vi "PH_Cam_BaseClass.set modified data.vi"(0 "i ref in":refnum<vi>, 2 "i attribute":T1={"Gui Refs"={"Frame Rate"=refnum, "Get Frame Rate"=refnum, "Show Image"=refnum, "Get Histogram"=refnum, "Mapping"=refnum, "Histogram"=refnum, "Center Cross"=refnum, "Center of Gravity"=refnum, "Scale Factor [%]"=refnum, "Save Image"=refnum, "Palette"=refnum, "Subtract Background"=refnum, "Cam Error"=refnum, "On"=refnum, "Cam List"=refnum}, "Cam"={"Source Notifier"=refnum, "Error"={"status"=FALSE, "code"=0, "source"=""}, "Camera ID"="N/A"}, "Images"={"Cam"=refnum, "Operation"=refnum, "PSDB"=refnum}, "Window Image"={"Indicate Image"=FALSE, "Window No."=0, "Scale Facor"=0.5, "Center Cross"=FALSE, "Subtract Backgr"=FALSE, "CoG"=FALSE, "Color Palette"=[], "Image On"=FALSE}, "Default Prdc Int"=50, "Performance"={"on"=FALSE, "Timestamp Last Frame"=0}, "Histogram"={"on"=FALSE, "Mapping"=FALSE}, "Save Image"={"Save"=FALSE, "File refnum"=refnum}, "Setting Service ID"=0, "Screen"={"x-resolution"=0, "y-resolution"=0}, "On"=FALSE, "Constructor finished"=FALSE, "configured"=FALSE} {"Cam"."Error"."code" format="%.0x"}, 5 "error in (no error)":errorcluster) -> (14 "i ref out":refnum<vi>, 19 "error out":errorcluster)   [LabVIEW 2014, in "PH_Cam_BaseClass.lvlib"]
doc: "Writes the data into the attribute of an object. Then, the attribute dara are unlocked using the \"release\" method. Prior to calling THIS method, the attribute data must have been locked using the methods \"lock\" or \"get data to modify\".\n\n\nLicense Agreement for this software:\n\nCopyright (C)\nGesellschaft für Schwerionenforschung, GSI\nPlanckstr. 1\n64291 Darmstadt\nGermany\n\nContact: D.Beck@gsi.de \n\nThis program is free software; you can redistribute it and/or modify it under the terms of the GNU General Public License as published by the Free Software Foundation; either version 2 of the license, or (at your option) any later version.\n\nThis program is distributed in the hope that it will be useful, but WITHOUT ANY WARRANTY; without even the implied warranty of MERCHANTABILITY or FITNESS FOR A PARTICULAR PURPOSE. See the GNU General License for more details (http://www.gnu.org).\n\nGesellschaft für Schwerionenforschung, GSI\nPlanckstr. 1, 64291 Darmstadt, Germany\nFor all questions and ideas contact: M.Richter@gsi.de, H.Brand@gsi.de or D.Beck@gsi.de.\nLast update: 17-JUN-2004"
uses:
  PH_Cam_BaseClass.lvlib
  PH_Cam_BaseClass.i attribute.ctl
  PH_Cam_BaseClass.GUI Refs.ctl
  <vilib>/vision/Image Controls.llb/IMAQ Image.ctl
  CSCore/CSObj/CSObj.lvlib
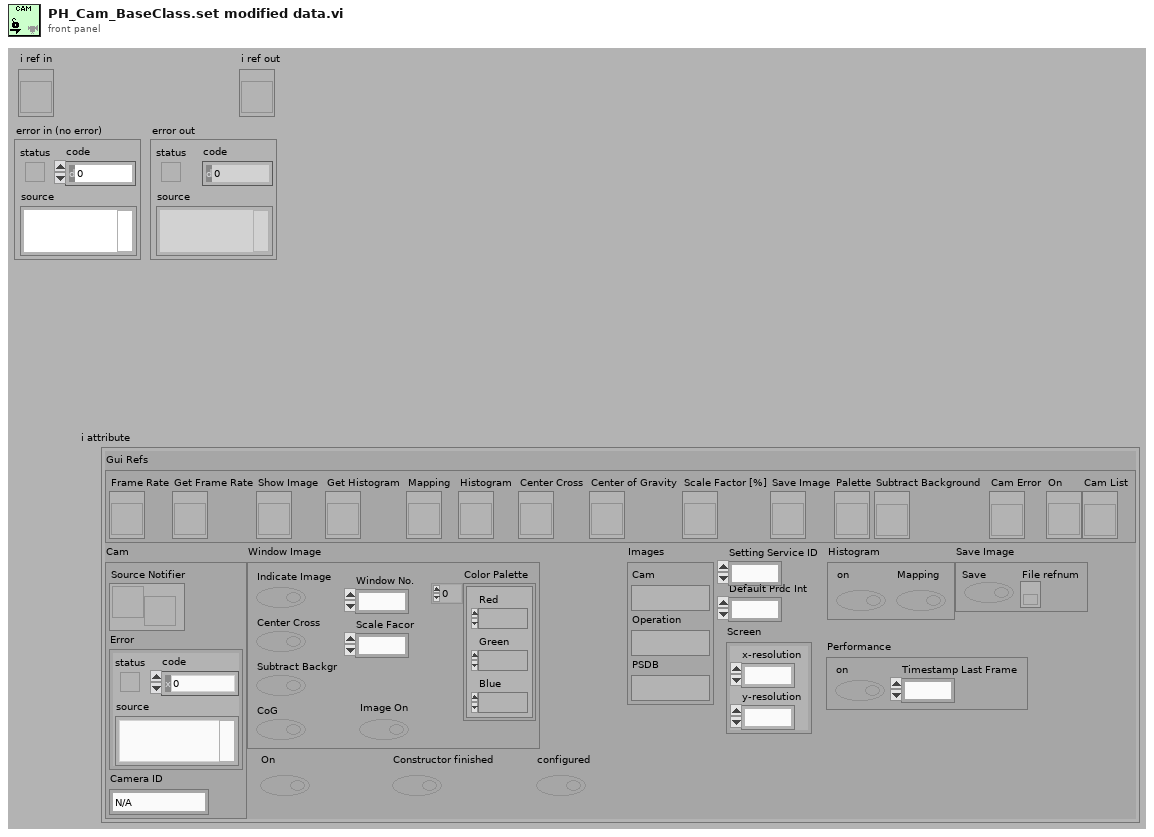
[diagram p1: front panel]
types:
  T1 = typedef "PH_Cam_BaseClass.lvlib/PH_Cam_BaseClass.i attribute.ctl" = cluster{"Gui Refs":T2, "Cam":cluster{"Source Notifier":refnum<notifier>, "Error":errorcluster, "Camera ID":string}, "Images":cluster{"Cam":T3, "Operation":T3, "PSDB":T3}, "Window Image":cluster{"Indicate Image":bool, "Window No.":i32, "Scale Facor":dbl, "Center Cross":bool, "Subtract Backgr":bool, "CoG":bool, "Color Palette":cluster{"Red":u8, "Green":u8, "Blue":u8}[], "Image On":bool}, "Default Prdc Int":i32, "Performance":cluster{"on":bool, "Timestamp Last Frame":i32}, "Histogram":cluster{"on":bool, "Mapping":bool}, "Save Image":cluster{"Save":bool, "File refnum":refnum<file>}, "Setting Service ID":i32, "Screen":cluster{"x-resolution":i16, "y-resolution":i16}, "On":bool, "Constructor finished":bool, "configured":bool}
  T2 = typedef "PH_Cam_BaseClass.lvlib/PH_Cam_BaseClass.GUI Refs.ctl" = cluster{"Frame Rate":refnum<vi>, "Get Frame Rate":refnum<vi>, "Show Image":refnum<vi>, "Get Histogram":refnum<vi>, "Mapping":refnum<vi>, "Histogram":refnum<vi>, "Center Cross":refnum<vi>, "Center of Gravity":refnum<vi>, "Scale Factor [%]":refnum<vi>, "Save Image":refnum<vi>, "Palette":refnum<vi>, "Subtract Background":refnum<vi>, "Cam Error":refnum<vi>, "On":refnum<vi>, "Cam List":refnum<vi>}
  T3 = typedef "IMAQ Image.ctl" = refnum<image>
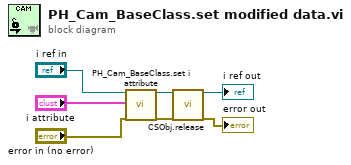
[diagram p0: block diagram]
diagram:
  n1 = call "PH_Cam_BaseClass.set i attribute.vi"("i ref in"="i ref in", "i attribute"="i attribute", "error in (no error)"="error in (no error)") -> ("i ref out"=w4:refnum<vi>, "error out"=w3:errorcluster)  [unwired: 15 in]
  n2 = call "CSObj.release.vi"("i ref in"=w4, "error in (no error)"=w3) -> ("i ref out"=→"i ref out":refnum<vi>, "error out"=→"error out":errorcluster)  [unwired: 16 in]
